vi "metniseseçevirme.vi"() -> ()   [LabVIEW 2017]
uses:
  System.Speech
panel:
  in  "Durdur":bool
  out "Metin Belgesi":string
  in  "Dosya Seçiniz":path
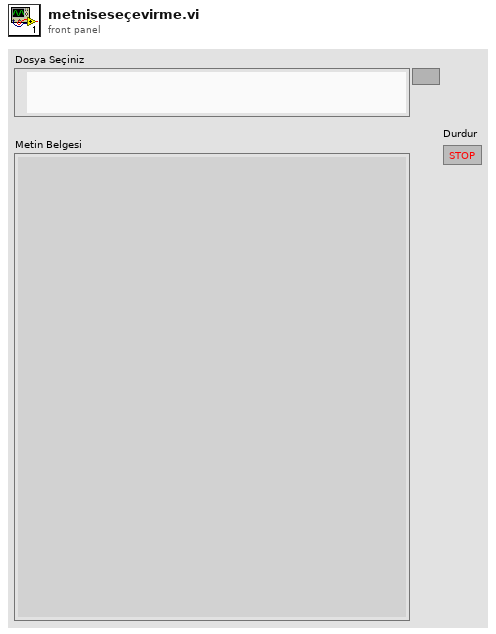
[diagram p1: front panel]
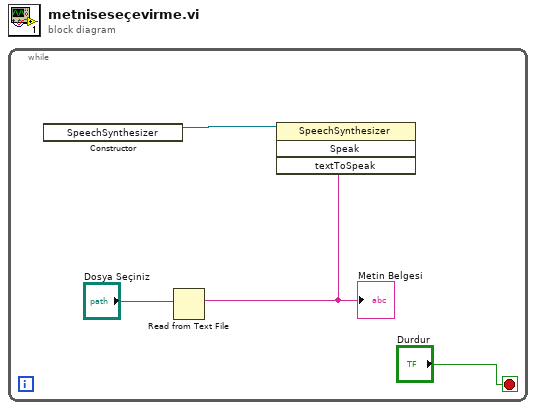
[diagram p0: block diagram]
diagram:
  n1 = while {
    stop <- "Durdur" stop-if-true
    n2 = constructor class="SpeechSynthesizer"() -> (reference out=w2:refnum<k24>)  [unwired: 3 in, 2 out]
    n3 = Read from Text File(file (use dialog)="Dosya Seçiniz") -> (text=w4:string)  [unwired: 3 in, 3 out]
    "Metin Belgesi" <- w4
    n4 = invoke class="SpeechSynthesizer" method="Speak"(reference=w2, "textToSpeak"=w4) -> ()  [unwired: 2 in, 4 out]
  }
